vi "Generate Waveforms.vi"(1 "Single Tone.lvclass":refnum<class "Silence.lvclass">) -> (0 "Waveforms":waveform(dbl)[](array[waveform]))   [LabVIEW 2010, in "Silence.lvclass"]
uses:
  Silence.lvclass
  Silence.lvclass/Silence.ctl
  <vilib>/measure/NI_MABase.lvlib
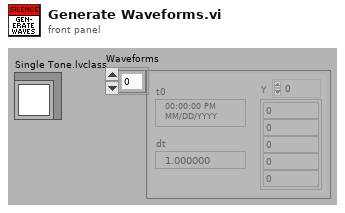
[diagram p1: front panel]
types:
  T1 = cluster{"Samples per second":dbl, "Number of samples":dbl}
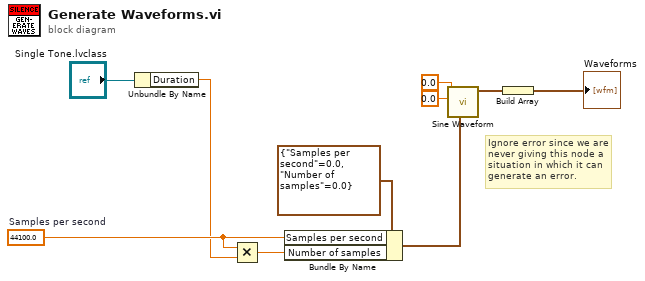
[diagram p0: block diagram]
diagram:
  w6 = 44100.0  # Samples per second
  # "Ignore error since we are\nnever giving this node a\nsituation in which it can\ngenerate an error."
  n1 = Unbundle By Name("Single Tone.lvclass") -> ("Duration"=w5:dbl)
  n2 = Multiply(x=w6, y=w5) -> (x*y=w7:dbl)
  n3 = Bundle By Name(cluster=T1 {"Samples per second"=0.0, "Number of samples"=0.0} ("sampling info"), "Samples per second"=w6, "Number of samples"=w7) -> (w4:T1)
  n4 = call <vilib>:"Sine Waveform.vi"("sampling info"=w4, "amplitude"=0.0, "frequency"=0.0) -> ("signal out"=w3:waveform(dbl))  [unwired: 7 in, 1 out]
  n5 = Build Array(w3) -> (→"Waveforms":waveform(dbl)[])
